vi "Read Main Path.vi"(8 "error in":errorcluster, 11 "System Log in":refnum<class "System Log.lvclass">) -> (0 "error out":errorcluster, 2 "Main Path":path, 3 "System Log out":refnum<class "System Log.lvclass">)   [LabVIEW 2014, in "System Log.lvclass"]
uses:
  System Log.lvclass
  System Log.lvclass/System Log.ctl
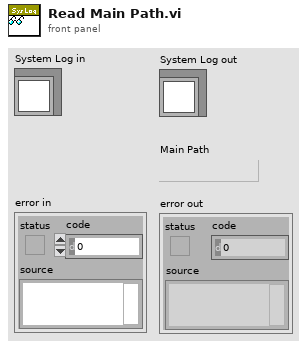
[diagram p1: front panel]
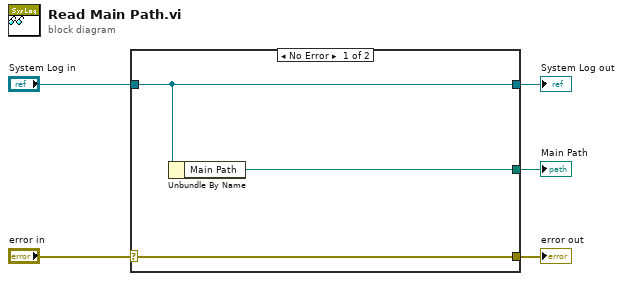
[diagram p0: block diagram]
diagram:
  n1 = case shown="No Error" "error in" {
    selector: "error in" -> [w8 w9]
    tunnel: [w8 w9] -> w4
    tunnel: [w7 w10] -> w2
    tunnel: "System Log in" -> [w7 w10]
    tunnel: [w6 _] -> w1
    frame No Error {
      n2 = Unbundle By Name(w7) -> ("Main Path"=w6:path)
    }
    frame Error {
    }
  }
  "error out" <- w4
  "System Log out" <- w2
  "Main Path" <- w1
